vi "Format Step Tag.vi"(11 "Step Number":i32) -> (3 "Tag":string)   [LabVIEW 2020, in "Output Sequencer.lvlib" / "Settings UI.lvclass"]
uses:
  Settings UI.lvclass
  Types/Tree Index Enum.ctl
  Globals/Global Tree Data.vi
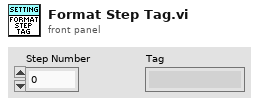
[diagram p1: front panel]
types:
  T1 = typedef "Output Sequencer.lvlib/Settings UI.lvclass/Tree Index Enum.ctl" = enum16{"General Settings", "Num Steps", "Num Analog", "Num Digital", "Show Confirmation", "Interp Priority", "Adv Timing", "Enable Conditions", "Seq Execution", "Reset Test Start", "Only When Test", "Delay After Test", "Start condition", "Re-triggering", "Stop condition", "Stop After Cycles", "Stop Values", "Default Values", "Default Analog", "Default Digital", "Steps", "Step #", "Description", "Precondition", "Duration", "Mode", "Delay Between Vals", "Analog Values", "Digital Values", "Postcondition", "On True", "On False"}
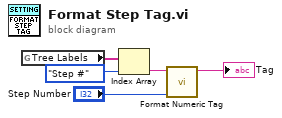
[diagram p0: block diagram]
diagram:
  n1 = global read "Global Tree Data.vi" "Tree Labels"() -> (w1:string[])
  n2 = Index Array(array=w1, index=Tree_Index_Enum."Step #" ("Tree Index Enum")) -> (element=w3:string)
  n3 = call "Format Numeric Tag.vi"("Number"="Step Number", "Tree label"=w3) -> ("Tag"=→"Tag":string)  [unwired: 9 in]
